vi "Write to Source.vi"(11 "value":dbl) -> (0 "error out":errorcluster)   [LabVIEW 2013]
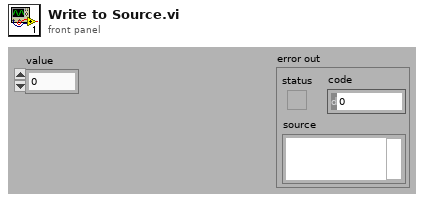
[diagram p1: front panel]
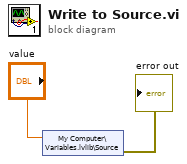
[diagram p0: block diagram]
diagram:
  n1 = shared-variable "My Computer\\Variables.lvlib\\Source"("value") -> (error out=→"error out":errorcluster)  [unwired: 1 out]
